vi "WPI_CANTalonSRX_MotionProfile_IterateFlowControl.vi"(9 "Is F(x)":bool, 10 "Input":i32) -> (2 "Output":i32)   [LabVIEW 2016]
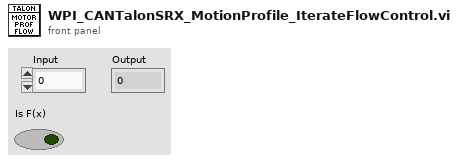
[diagram p1: front panel]
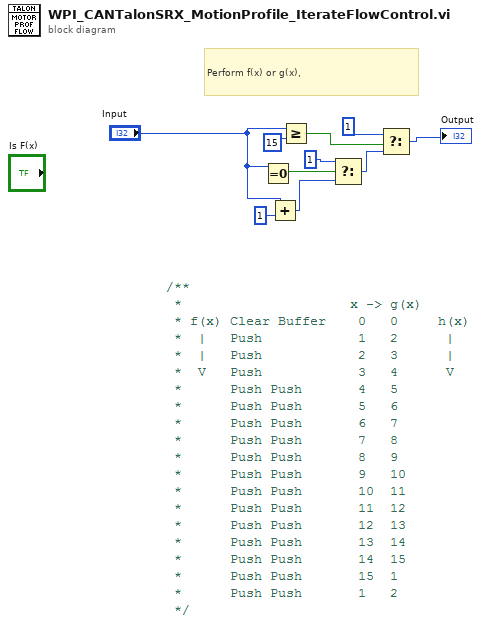
[diagram p0: block diagram]
diagram:
  # "Perform f(x) or g(x),"
  n1 = Equal To 0?(x="Input") -> (x = 0?=w6:bool)
  n2 = Add(x="Input", y=u8 1) -> (x+y=w4:i32)
  n3 = Greater Or Equal?(x="Input", y=u8 15) -> (x >= y?=w8:bool)
  n4 = Select(t=u32 1, s=w6, f=w4) -> (s? t:f=w3:u32)
  n5 = Select(t=u8 1, s=w8, f=w3) -> (s? t:f=→"Output":u32)
